vi "Set BG Image.vi"(8 "error in (no error)":errorcluster, 11 "HIJ Vision Camera App in":refnum<class "HIJ Vision Camera App.lvclass">) -> (0 "error out":errorcluster, 2 "BG image path":path, 3 "HIJ Vision Camera App out":refnum<class "HIJ Vision Camera App.lvclass">)   [LabVIEW 2020, in "HIJ Vision Camera App.lvlib" / "HIJ Vision Camera App.lvclass"]
uses:
  HIJ Vision Camera App.lvclass
  C:/Users/AlexK/work/LabVIEW Programme/POLARIS CAM Log Abw und E/Submodules/HIJ Vision/Application Base Actors/HIJ Vision Application/HIJ Vision Application/HIJ Vision Application.lvclass
  HIJ Vision Application/HIJ Vision Application/HIJ Vision Application.lvclass/HIJ Vision Application.ctl
  <vilib>/ActorFramework/Message Enqueuer/Message Enqueuer.lvclass/Message Enqueuer.ctl
  HIJ Vision Application/HIJ Vision Application/Read Display Enq.vi
  <vilib>/ActorFramework/Message Enqueuer/Enqueue.vi
  Display Actors/HIJ IMAQdx Display/AF IMAQ Display Messages/Write BG Image Msg/Set BG Image Msg.lvclass
  C:/Program Files (x86)/National Instruments/LabVIEW 2020/vi.lib/ActorFramework/Message/Message.lvclass
  <vilib>/ActorFramework/Message Priority Queue/Priority Enqueue.vi
  <vilib>/ActorFramework/Message Enqueuer/Message Enqueuer.lvclass
  HIJ Vision Camera App.lvclass/HIJ Vision Camera App.ctl
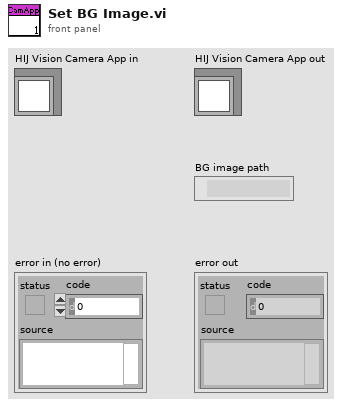
[diagram p1: front panel]
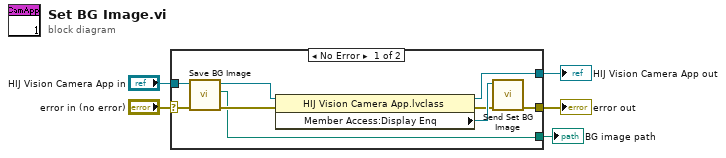
[diagram p0: block diagram]
diagram:
  n1 = case shown="No Error" "error in (no error)" {
    selector: "error in (no error)" -> [w8 w16]
    tunnel: [w12 w16] -> w4
    tunnel: [w10 w15] -> w2
    tunnel: "HIJ Vision Camera App in" -> [w11 w15]
    tunnel: [w6 _] -> w1
    frame No Error {
      n2 = call-dynamic "Save BG Image.vi"("error in (no error)"=w8, "HIJ Vision Camera App In"=w11) -> ("error out"=w7:errorcluster, "image path"=w6:path, "HIJ Vision Camera App Out"=w9:refnum<class "HIJ Vision Camera App.lvclass">)  [unwired: 7 in]
      n3 = property class="HIJ Vision Camera App.lvclass"(reference=w9, error in=w7) -> (reference out=w10:refnum<class "HIJ Vision Camera App.lvclass">, error out=w13:errorcluster, "Member Access:Display Enq"=w14:refnum<class "Message Enqueuer.lvclass">)
      n4 = call "Send Set BG Image.vi"("error in (no error)"=w13, "Message Enqueuer"=w14) -> ("error out"=w12:errorcluster)  [unwired: 8 in, 1 out]
    }
    frame Error {
    }
  }
  "error out" <- w4
  "HIJ Vision Camera App out" <- w2
  "BG image path" <- w1
